vi "GetColor.vi"(8 "error in (no error)":errorcluster, 11 "ColorRGBA in":refnum<class "ColorRGBA.lvclass">) -> (0 "error out":errorcluster, 2 "Color":u32(colorbox), 3 "ColorRGBA out":refnum<class "ColorRGBA.lvclass">)   [LabVIEW 2021, in "Picture2D.lvlib" / "ColorRGBA.lvclass"]
uses:
  ColorRGBA.lvclass
  ColorRGBA.lvclass/ColorRGBA.ctl
  ColorRGB/ColorRGB.lvclass
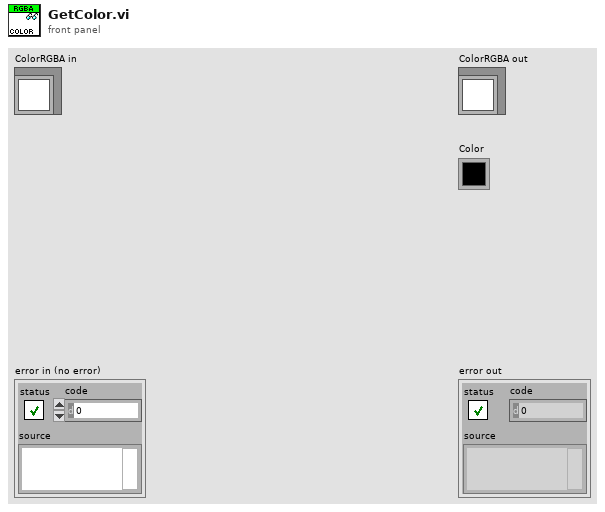
[diagram p1: front panel]
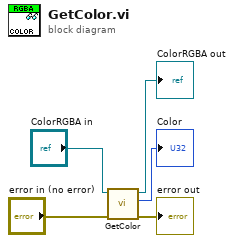
[diagram p0: block diagram]
diagram:
  n1 = call-parent "GetColor.vi"("error in (no error)"="error in (no error)", "ColorRGB in"="ColorRGBA in") -> ("error out"=→"error out":errorcluster, "Color"=→"Color":u32, "ColorRGB out"=→"ColorRGBA out":refnum<class "ColorRGBA.lvclass">)  [unwired: 7 in]
